vi "VI Server_Get_INI_FilePath.vi"(8 "error in (no error)":errorcluster, 11 "VI Server Cluster":T1) -> (0 "error out":errorcluster, 2 "INI File Path":path, 3 "VI Server Cluster.DUP":T1)   [LabVIEW 2020, in "VI Server Toolkit LV2013.lvlib"]
doc: "Generates an INI file path in reference to the calling VI."
uses:
  VI Server Toolkit LV2013.lvlib
  VI Server_TypeDefs/VI Server_RefsCluster.ctl
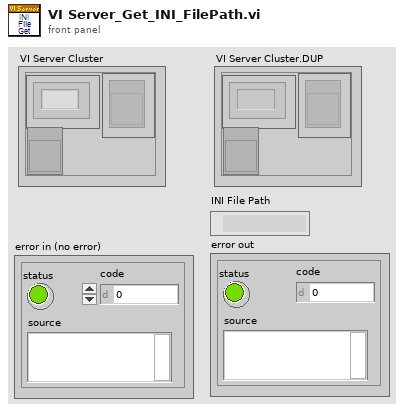
[diagram p1: front panel]
types:
  T1 = typedef "VI Server_RefsCluster.ctl" = cluster{"Labels":string[], "Refs":refnum<vi>[], "VI Ref":refnum<vi>}
  T2 = enum32{"invalid app kind", "Development System", "Run Time System", "Student Edition", "Embedded LabVIEW", "Evaluation", "Custom"}
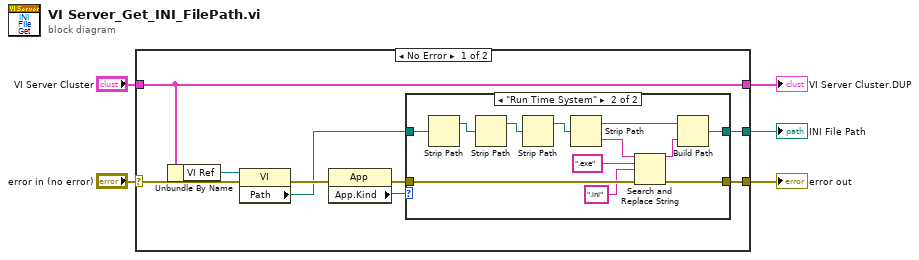
[diagram p0: block diagram]
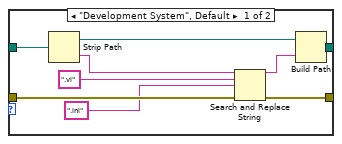
[diagram p2: hidden frame]
diagram:
  n1 = case shown="No Error" "error in (no error)" {
    selector: "error in (no error)" -> [w8 w36]
    tunnel: [w14 w36] -> w5
    tunnel: "VI Server Cluster" -> [w7 _]
    tunnel: [w9 _] -> w3
    tunnel: [w7 _] -> w1
    frame No Error {
      n2 = Unbundle By Name(w7) -> ("VI Ref"=w10:refnum<vi>)
      n3 = property class="VI"(reference=w10, error in=w8) -> (error out=w11:errorcluster, "Path"=w6:path)  [unwired: 1 out]
      n4 = property class="App"(error in=w11) -> (error out=w13:errorcluster, "App.Kind"=w12:T2)  [unwired: 1 in, 1 out]
      n5 = case shown="\"Run Time System\"" w12 {
        tunnel: w13 -> [w22 w35]
        tunnel: [w21 w34] -> w14
        tunnel: w6 -> [w23 w29]
        tunnel: [w15 w30] -> w9
        frame "Development System", Default {
          n6 = Strip Path(path=w23) -> (stripped path=w17:path, name=w20:string)
          n7 = Search and Replace String(input string=w20, search string=".vi", replace string=".ini" ("replace string (\"\")"), error in=w22) -> (result string=w16:string, error out=w21:errorcluster)  [unwired: 4 in, 2 out]
          n8 = Build Path(base path=w17, name or relative path=w16) -> (appended path=w15:path)
        }
        frame "Run Time System" {
          n9 = Strip Path(path=w29) -> (stripped path=w28:path)  [unwired: 1 out]
          n10 = Strip Path(path=w28) -> (stripped path=w25:path)  [unwired: 1 out]
          n11 = Strip Path(path=w25) -> (stripped path=w24:path)  [unwired: 1 out]
          n12 = Strip Path(path=w24) -> (stripped path=w27:path, name=w26:string)
          n13 = Search and Replace String(input string=w26, search string=".exe", replace string=".ini" ("replace string (\"\")"), error in=w35) -> (result string=w31:string, error out=w34:errorcluster)  [unwired: 4 in, 2 out]
          n14 = Build Path(base path=w27, name or relative path=w31) -> (appended path=w30:path)
        }
      }
    }
    frame Error {
    }
  }
  "error out" <- w5
  "VI Server Cluster.DUP" <- w1
  "INI File Path" <- w3
